vi "User GFV ini.vi"(1 "Action(GET)":T1(ring), 7 "User ID in":T2, 11 "error in (no error)":errorcluster) -> (8 "User ID out":T2, 15 "error out":errorcluster)   [LabVIEW 2011]
uses:
  User Indikator.ctl
  Super User bool indikator.ctl
  <vilib>/Utility/VariantDataType/VariantType.lvlib
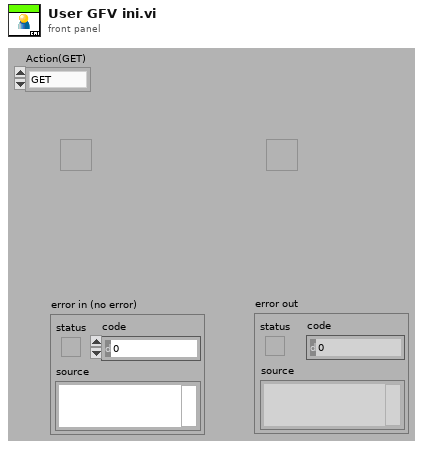
[diagram p1: front panel]
types:
  T1 = enum16{"GET", "SET", "Get from Ini", "Put in Ini"}
  T2 = typedef "User Indikator.ctl" = cluster{"User Name":string, "Super User":T3}
  T3 = typedef "Super User bool indikator.ctl" = bool
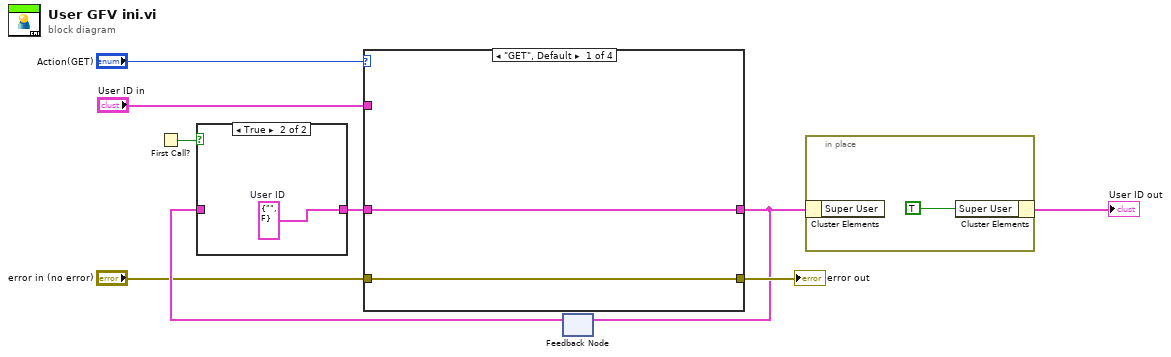
[diagram p0: block diagram]
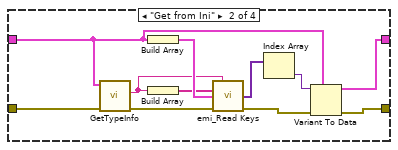
[diagram p3: hidden frame]
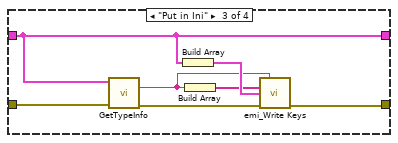
[diagram p4: hidden frame]
diagram:
  n1 = First Call?() -> (First Call?: T/F=w8:bool)
  n2 = feedback #1() -> (w9:T2)  [unwired: 1 in]
  n3 = case shown="True" w8 {
    tunnel: w9 -> [w10 _]
    tunnel: [w10 w11] -> w7
    frame False {
    }
    frame True {
      w11 = T2 {"User Name"="", "Super User"=FALSE}  # User ID
    }
  }
  n4 = case shown="\"GET\", Default" "Action(GET)" {
    tunnel: [w13 w14 w25 w33] -> w2
    tunnel: w7 -> [w13 w15 w25 _]
    tunnel: "User ID in" -> [_ _ _ w33]
    tunnel: "error in (no error)" -> [w12 w19 w27 w32]
    tunnel: [w12 w17 w26 w32] -> w3
    frame "GET", Default {
    }
    frame "Get from Ini" {
      n5 = call <vilib>:"GetTypeInfo.vi"("error in (no error)"=w19, "Variant"=w15) -> ("error out"=w23:errorcluster, "Name"=w21:string)  [unwired: 5 in, 3 out]
      n6 = Build Array(w15) -> (w24:T2[])
      n7 = Build Array(w21) -> (w22:string[])
      n8 = call "emi_Read Keys.vi"("Section"=w21, "Key Names"=w22, "Types/Defaults"=w24, "error in (no error)"=w23) -> ("Values"=w20:variant[], "error out"=w18:errorcluster)  [unwired: 9 in, 1 out]
      n9 = Index Array(array=w20) -> (element=w16:variant)  [unwired: 1 in]
      n10 = Variant To Data(error in=w18, type=w15, Variant=w16) -> (data=w14:T2, error out=w17:errorcluster)
    }
    frame "Put in Ini" {
      n11 = call <vilib>:"GetTypeInfo.vi"("error in (no error)"=w27, "Variant"=w25) -> ("error out"=w30:errorcluster, "Name"=w28:string)  [unwired: 5 in, 3 out]
      n12 = Build Array(w25) -> (w31:T2[])
      n13 = Build Array(w28) -> (w29:string[])
      n14 = call "emi_Write Keys.vi"("Section"=w28, "Key Names"=w29, "Values"=w31, "error in (no error)"=w30) -> ("error out"=w26:errorcluster)  [unwired: 10 in, 1 out]
    }
    frame "SET" {
    }
  }
  "error out" <- w3
  n15 = feedback-in #1(w2) -> ()
  n16 = in-place {
    n17 = in-place-cluster #2(w2) -> ()  [unwired: 1 out]
    n18 = in-place-cluster #2("Super User"=T3 TRUE) -> (→"User ID out":T2)
  }
